vi "pause1.vi"() -> ()   [LabVIEW 2020]
panel:
  in  "pause1":bool
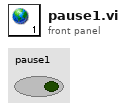
[diagram p1: front panel]
diagram:
